vi "JKI Arguments Used.vi"(8 "error in":errorcluster, 11 "CaseSel Refnum":refnum<vi>) -> (0 "error out":errorcluster, 3 "Arguments used?":bool)   [LabVIEW 2020]
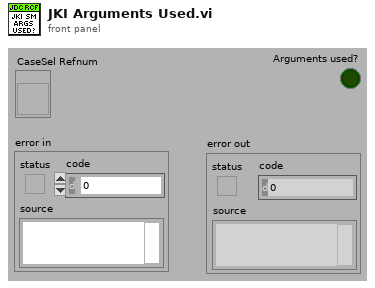
[diagram p1: front panel]
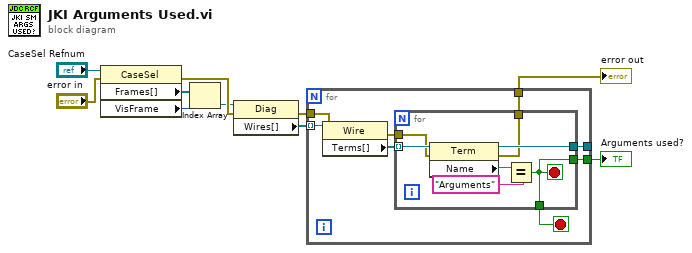
[diagram p0: block diagram]
diagram:
  n1 = property class="CaseSel"(reference="CaseSel Refnum", error in="error in") -> (error out=w10:errorcluster, "Frames[]"=w6:refnum<vi>[], "VisFrame"=w5:u32)  [unwired: 1 out]
  n2 = Index Array(array=w6, index=w5) -> (element=w2:refnum<vi>)
  n3 = property class="Diag"(reference=w2, error in=w10) -> (error out=w9:errorcluster, "Wires[]"=w4:refnum<vi>[])  [unwired: 1 out]
  n4 = for {
    tunnel: w4 -> [w17] mode=indexing
    tunnel: [w16] -> _
    tunnel: [w14] -> w1
    tunnel: [w13] -> w8
    tunnel: w9 -> [w11]
    stop <- w15 stop-if-true
    n5 = property class="Wire"(reference=w17, error in=w11) -> (error out=w12:errorcluster, "Terms[]"=w18:refnum<vi>[])  [unwired: 1 out]
    n6 = for {
      tunnel: w18 -> [w25] mode=indexing
      tunnel: [w23] -> w16
      tunnel: [w21] -> w15
      tunnel: [w21] -> w14
      tunnel: [w20] -> w13
      tunnel: w12 -> [w19]
      stop <- w21 stop-if-true
      n7 = property class="Term"(reference=w25, error in=w19) -> (reference out=w23:refnum<vi>, error out=w20:errorcluster, "Name"=w22:string)
      n8 = Equal?(x=w22, y="Arguments") -> (x = y?=w21:bool)
    }
  }
  "Arguments used?" <- w1
  "error out" <- w8
